vi "AddArea.vi"(4 "Size":u8, 6 "Value":u32, 8 "Yloc":u32, 9 "Xloc":u32, 11 "ArrayIn":u32[][](array[numeric])) -> (3 "ArrayOut":u32[][](array[numeric]))   [LabVIEW 2014]
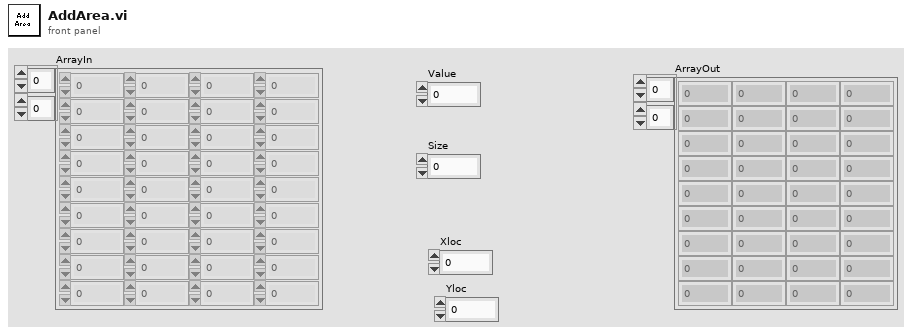
[diagram p1: front panel]
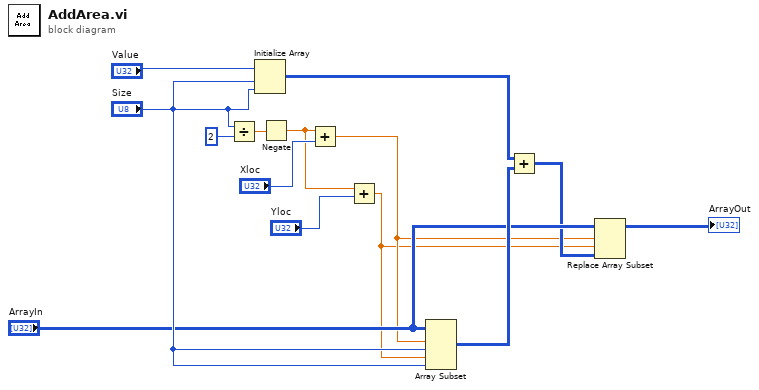
[diagram p0: block diagram]
diagram:
  n1 = Divide(x="Size", y=u8 2) -> (x/y=w12:dbl)
  n2 = Initialize Array("Value", "Size", "Size") -> (w7:u32[][])
  n3 = Negate(x=w12) -> (-x=w10:dbl)
  n4 = Add(x=w10, y="Xloc") -> (x+y=w3:dbl)
  n5 = Add(x=w10, y="Yloc") -> (x+y=w2:dbl)
  n6 = Array Subset(array="ArrayIn", index (row)=w3, length (row)="Size", index (col)=w2, length (col)="Size") -> (w6:u32[][])
  n7 = Add(x=w7, y=w6) -> (x+y=w4:u32[][])
  n8 = Replace Array Subset(array="ArrayIn", new element=w4, index (row)=w3, index (col)=w2) -> (→"ArrayOut":u32[][])
